vi "Carbon - Setup Mega.vi"(8 "error in (no error)":errorcluster, 10 "Password":string, 11 "User@Session":string="cbuurma@mega ") -> (0 "error out":errorcluster, 3 "Error String":string)   [LabVIEW 2010]
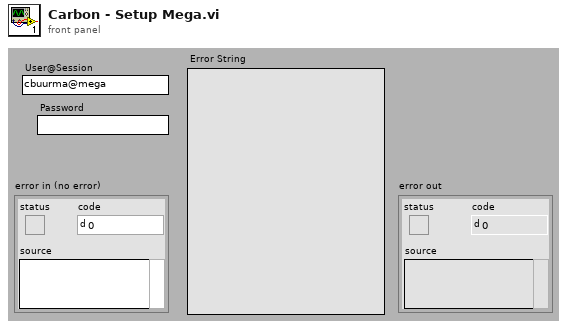
[diagram p1: front panel]
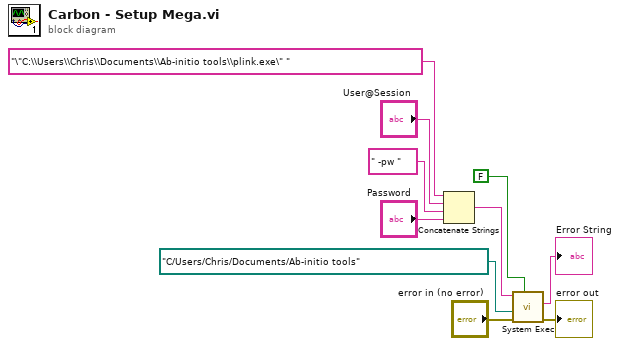
[diagram p0: block diagram]
diagram:
  n1 = Concatenate Strings("\"C:\\Users\\Chris\\Documents\\Ab-initio tools\\plink.exe\" ", "User@Session", " -pw ", "Password") -> (w9:string)
  n2 = call <vilib>:"System Exec.vi"("wait until completion? (T)"=FALSE, "error in (no error)"="error in (no error)", "working directory"=path "C:/Users/Chris/Documents/Ab-initio tools", "command line"=w9) -> ("error out"=→"error out":errorcluster, "standard error"=→"Error String":string)  [unwired: 4 in, 2 out]
